vi "CH1_Comm_TCPIP_NEW_Tx.vi"() -> ()   [LabVIEW 2018]
uses:
  TCPIP/TCPIP.lvclass
  RxTx/RxTx.lvclass
panel:
  out "error out 2":errorcluster
  in  "RxTx.lvclass 2":refnum<class "RxTx.lvclass">
  in  "TCPIP.lvclass 2":refnum<class "TCPIP.lvclass">
  out "error out 5":errorcluster
  in  "Channel":u16=1
  in  "Remote port":u16=59041
  # "Channel 1 - TCPIP Communication"
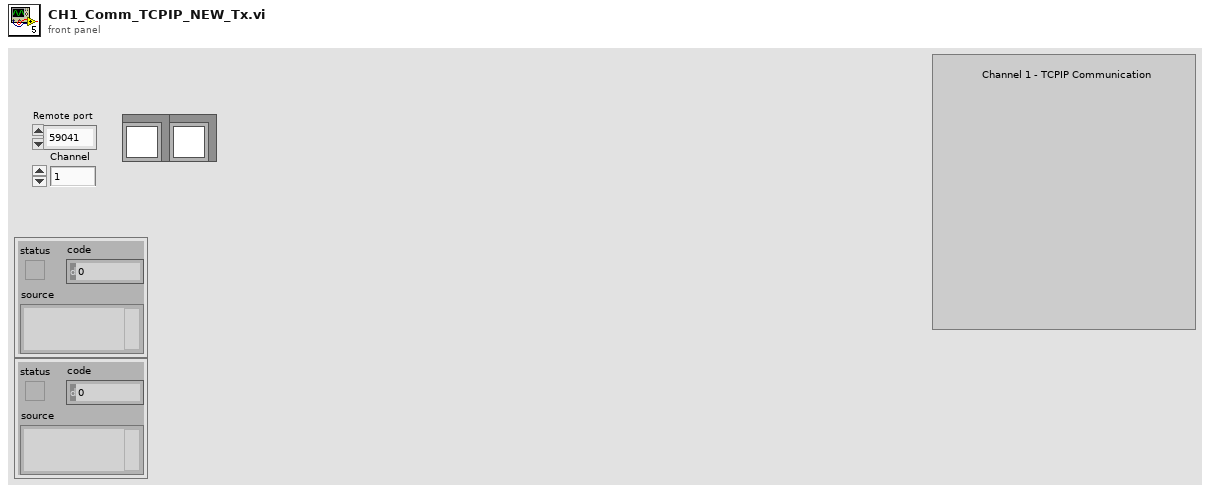
[diagram p1: front panel]
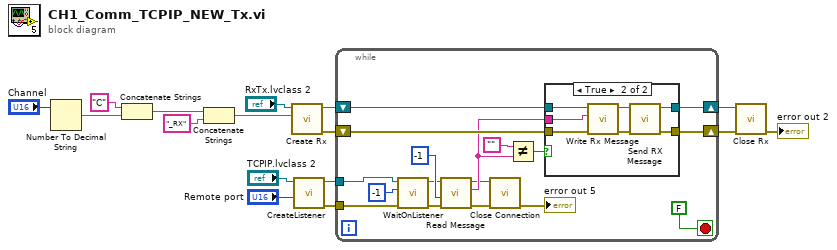
[diagram p0: block diagram]
diagram:
  n1 = Number To Decimal String(number="Channel") -> (decimal integer string=w13:string)  [unwired: 1 in]
  n2 = Concatenate Strings("C", w13) -> (w7:string)
  n3 = Concatenate Strings(w7, "_RX" ("Reader Name")) -> (w16:string)
  n4 = call "Create Rx.vi"("Reader Name"=w16, "RxTx in"="RxTx.lvclass 2") -> ("error out"=w11:errorcluster, "RxTx out"=w12:refnum<class "RxTx.lvclass">)  [unwired: 8 in]
  n5 = call-dynamic "CreateListener.vi"("remote port"="Remote port", "TCPIP in"="TCPIP.lvclass 2") -> ("error out"=w2:errorcluster, "TCPIP out"=w3:refnum<class "TCPIP.lvclass">)  [unwired: 8 in]
  n6 = while {
    shift-right: [w25] -> w9
    shift-left: w11 -> [w33]
    shift-right: [w26] -> w10
    shift-left: w12 -> [w32]
    tunnel: w3 -> [w24]
    tunnel: w2 -> [w21]
    stop <- FALSE stop-if-true
    n7 = call-dynamic "WaitOnListener.vi"("error in (no error)"=w21, "timeout ms"=-1, "TCPIP in"=w24) -> ("error out"=w20:errorcluster, "TCPIP out"=w27:refnum<class "TCPIP.lvclass">)  [unwired: 7 in]
    n8 = call "Read Message.vi"("error in (no error)"=w20, "timeout"=-1, "TCPIP in"=w27) -> ("error out"=w19:errorcluster, "Message"=w28:string, "TCPIP out"=w23:refnum<class "TCPIP.lvclass">)  [unwired: 6 in]
    n9 = call "Close Connection.vi"("error in (no error)"=w19, "TCPIP in"=w23) -> ("error out"=→"error out 5":errorcluster)  [unwired: 8 in, 1 out]
    n10 = Not Equal?(x="", y=w28) -> (x != y?=w30:bool)
    n11 = case shown="True" w30 {
      tunnel: w33 -> [w34 w40]
      tunnel: w32 -> [w35 w39]
      tunnel: [w35 w37] -> w26
      tunnel: [w34 w36] -> w25
      tunnel: w28 -> [_ w38]
      frame False {
      }
      frame True {
        n12 = call "Write Rx Message.vi"("error in (no error)"=w40, "Rx Message"=w38, "RxTx in"=w39) -> ("error out"=w41:errorcluster, "RxTx out"=w42:refnum<class "RxTx.lvclass">)  [unwired: 7 in]
        n13 = call "Send RX Message.vi"("error in (no error)"=w41, "RxTx in"=w42) -> ("error out"=w36:errorcluster, "RxTx out"=w37:refnum<class "RxTx.lvclass">)  [unwired: 8 in]
      }
    }
  }
  n14 = call "Close Rx.vi"("error in (no error)"=w9, "RxTx in"=w10) -> ("error out"=→"error out 2":errorcluster)  [unwired: 8 in, 1 out]
